vi "Read.vi"(0 "reference in":refnum<class "LCR_BK891.lvclass">, 11 "error in (no error)":errorcluster) -> (4 "reference in":refnum<class "LCR_BK891.lvclass">, 6 "Measured Primary Reading":dbl, 8 "Measured Secondary Reading":dbl, 15 "error out":errorcluster)   [LabVIEW 2022 SP3, in "LCR_BK891.lvlib" / "LCR_BK891.lvclass"]
uses:
  LCR_BK891.lvclass
  <vilib>/numeric/Random Number (Range) DBL.vi
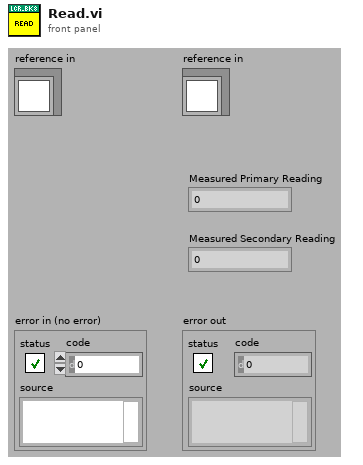
[diagram p1: front panel]
types:
  T1 = typedef "LCR_BK891.lvlib/LCR_BK891.lvclass/ObjectAttributes.ctl" = cluster{"Config":T2, "VISA Ref":refnum<visa-resource-name>, "Function":u16, "Range":u16, "Measurement Speed":u16, "Signal Frequency":dbl, "Signal Level":u8, "Measured Primary Reading":dbl, "Measured Secondary Reading":dbl}
  T2 = typedef "LCR_BK891.lvlib/LCR_BK891.lvclass/Config.ctl" = cluster{"VISA":refnum<visa-resource-name>}
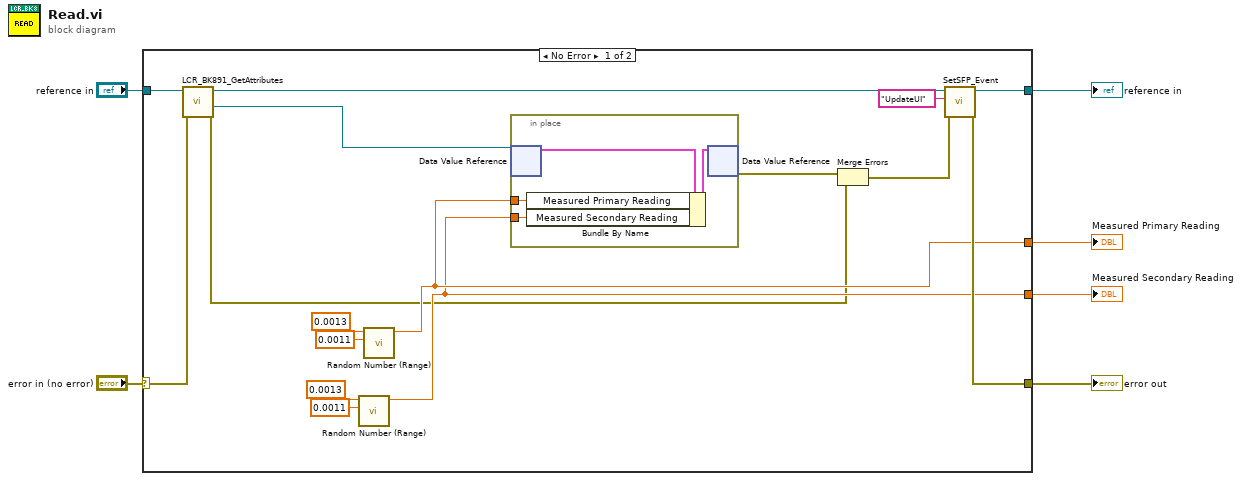
[diagram p0: block diagram]
diagram:
  n1 = case shown="No Error" "error in (no error)" {
    selector: "error in (no error)" -> [w22 w28]
    tunnel: [w17 w28] -> w5
    tunnel: [w18 w27] -> w3
    tunnel: "reference in" -> [w21 w27]
    tunnel: [w9 _] -> w2
    tunnel: [w8 _] -> w1
    frame No Error {
      n2 = call "LCR_BK891_GetAttributes.vi"("error in (no error)"=w22, "reference in"=w21) -> ("error out"=w7:errorcluster, "DataRef"=w20:refnum<data-value>, "reference out"=w19:refnum<class "LCR_BK891.lvclass">)  [unwired: 6 in, 1 out]
      n3 = call-poly <vilib>:"Random Number (Range).vi"("lower bound (0)"=0.0011, "upper bound (100)"=0.0013) -> ("number"=w8:dbl)  [unwired: 9 in]
      n4 = call-poly <vilib>:"Random Number (Range).vi"("lower bound (0)"=0.0011, "upper bound (100)"=0.0013) -> ("number"=w9:dbl)  [unwired: 9 in]
      n5 = in-place {
        in-place-border: w8 -> [w24]
        in-place-border: w9 -> [w23]
        n6 = in-place-dvr #1(w20) -> (w26:T1)  [unwired: 1 out]
        n7 = Bundle By Name(cluster=w26, "Measured Primary Reading"=w23, "Measured Secondary Reading"=w24) -> (w25:T1)
        n8 = in-place-dvr #1(w25) -> (w16:errorcluster)  [unwired: 1 out]
      }
      n9 = Merge Errors(w16, w7) -> (w15:errorcluster)
      n10 = call-dynamic "SetSFP_Event.vi"("error in (no error)"=w15, "msg"="UpdateUI", "reference in"=w19) -> ("error out"=w17:errorcluster, "reference out"=w18:refnum<class "LCR_BK891.lvclass">)  [unwired: 7 in]
    }
    frame Error {
    }
  }
  "error out" <- w5
  "reference in" <- w3
  "Measured Secondary Reading" <- w1
  "Measured Primary Reading" <- w2
